vi "zs_example.vi"() -> ()   [LabVIEW 2014]
uses:
  Robot_Position.ctl
panel:
  in  "停止":bool
  in  "输入簇":T1
  out "平面俯视图":T2(plugin-control)
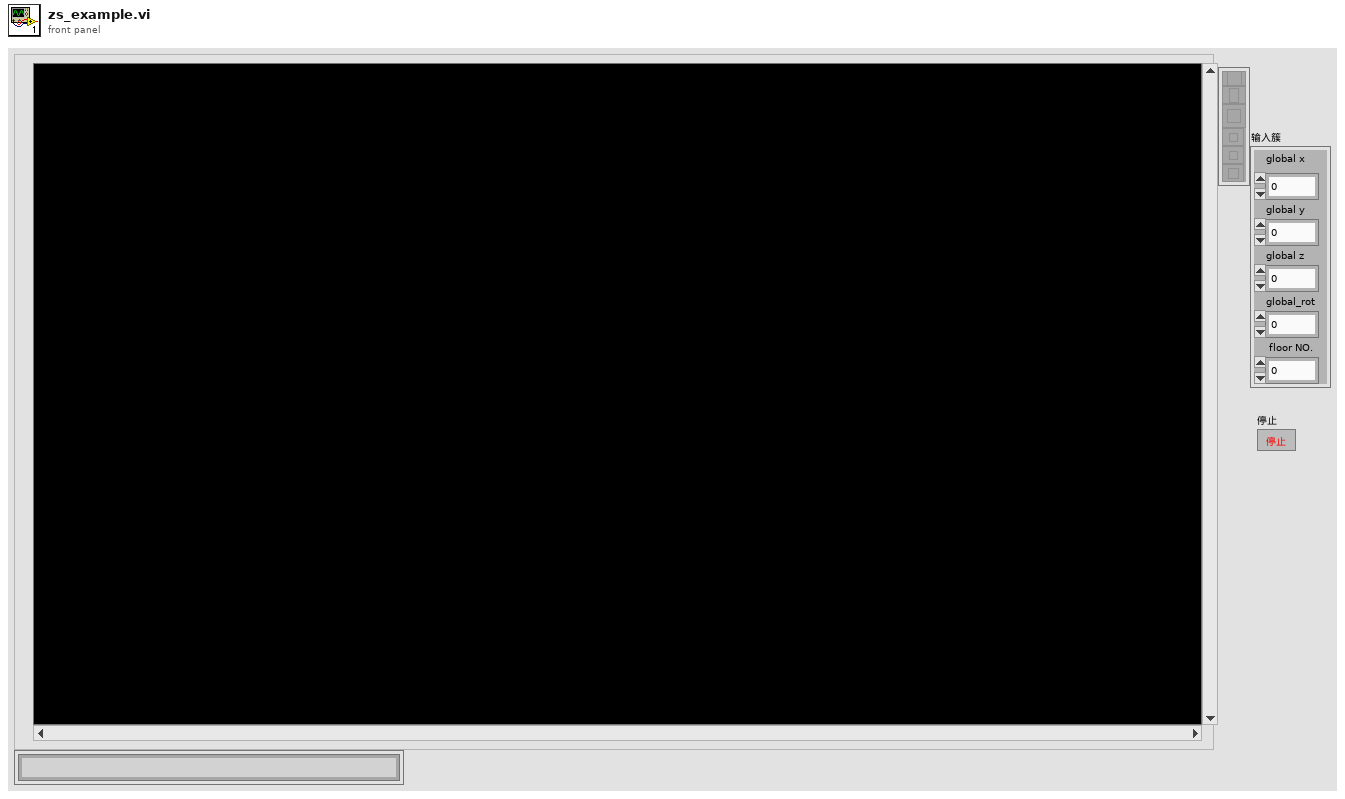
[diagram p1: front panel]
types:
  T1 = typedef "Robot_Position.ctl" = cluster{"global x":dbl, "global y":dbl, "global z":dbl, "global_rot":dbl, " floor NO.":dbl}
  T2 = typedef "IMAQ Image.ctl" = refnum<image>
  T3 = typedef "NI_Matrix.lvlib/RealMatrix.ctl" = dbl[][]
  T4 = cluster{"District Name":string, "Alias":string, "District Type":string, "Floor NO.":string, "Data Matrix":T3, "Path array":string[], "Path Coodinate":T3}[]
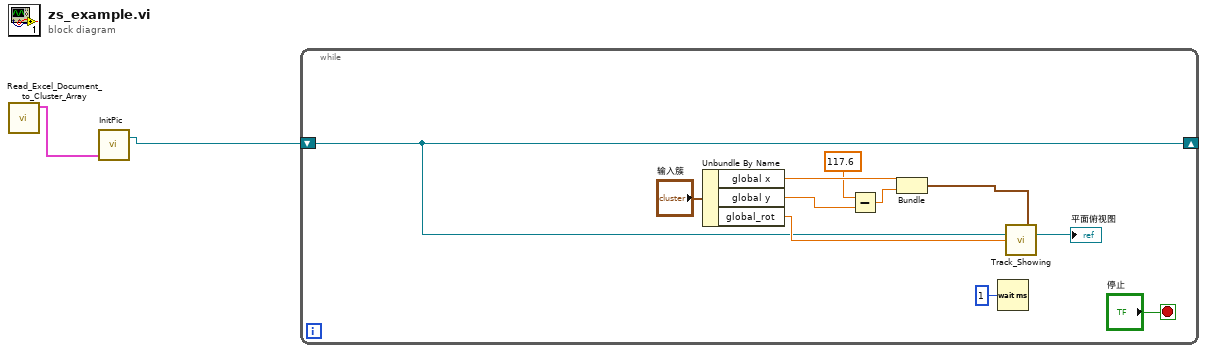
[diagram p0: block diagram]
diagram:
  n1 = call "Read_Excel_Document_to_Cluster_Array.vi"() -> ("Cluster of 7 Type Data_4F"=w1:T4)  [unwired: 7 in, 4 out]
  n2 = call "InitPic.vi"("Cluster of 7 Type Data"=w1) -> ("Image Out 2"=w2:T2)  [unwired: 3 in]
  n3 = while {
    shift-right: [w9] -> _
    shift-left: w2 -> [w9]
    stop <- "停止" stop-if-true
    n4 = Unbundle By Name("输入簇") -> ("global x"=w13:dbl, "global y"=w4:dbl, "global_rot"=w11:dbl)
    n5 = Subtract(x=117.6, y=w4) -> (x-y=w3:dbl)
    n6 = Bundle("global x"=w13, w3) -> (w6:cluster{"global x":dbl, dbl})  [unwired: 1 in]
    n7 = Wait (ms)(milliseconds to wait=u32 1 ("等待时间（毫秒）")) -> ()  [unwired: 1 out]
    n8 = call "Track_Showing.vi"("NewNodeM"=w6, "Image In 2"=w9, "数值"=w11) -> ("Image Out 2"=→"平面俯视图":T2)  [unwired: 12 in]
  }
